vi "generator.vi"() -> ()   [LabVIEW 2013]
panel:
  in  "dzialanie":u16(ring) items=["+", "-", "*", "/", ""]
  in  "z jakim?":u16(ring) items=["noise", "sin", "square", "sawtooth"]
  in  "jaki sygna³?":u16(ring) items=["noise", "sin", "square", "sawtooth"]
  out "wynik dzialania":waveform(dbl)(graph)
  in  "pocz.":dbl
  in  "amplituda":dbl=10.1 caption="Frequency"
  in  "krok":dbl=10.1 caption="Frequency"
  in  "próbkowanie":i32
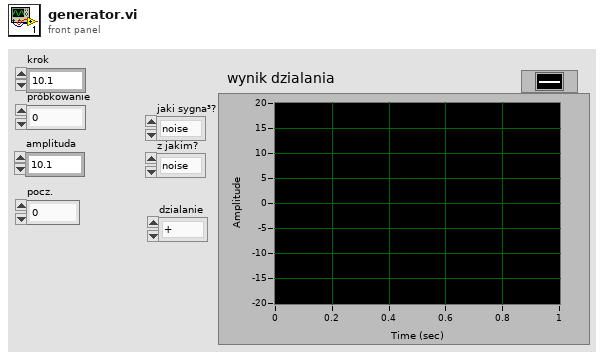
[diagram p1: front panel]
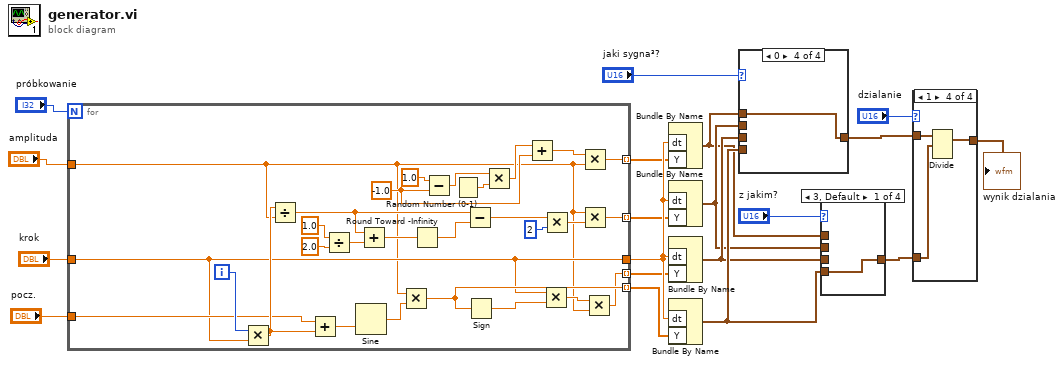
[diagram p0: block diagram]
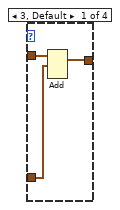
[diagram p2: hidden frame]
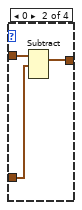
[diagram p3: hidden frame]
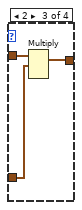
[diagram p4: hidden frame]
diagram:
  n1 = for {
    N: "próbkowanie" -> [_]
    tunnel: [w44] -> w14 mode=indexing
    tunnel: "krok" -> [w25]
    tunnel: [w47] -> w11 mode=indexing
    tunnel: [w21] -> w13 mode=indexing
    tunnel: "amplituda" -> [w20]
    tunnel: [w23] -> w12 mode=indexing
    tunnel: "pocz." -> [w26]
    tunnel: [w25] -> w15
    i -> [w43]
    w42 = -1.0 ("x")
    n2 = Multiply(x=w43, y=w25) -> (x*y=w27:dbl)
    n3 = Divide(x=w27, y=w20) -> (x/y=w34:dbl)
    n4 = Add(x=w26, y=w27) -> (x+y=w28:dbl)
    n5 = Divide(x=1.0, y=2.0) -> (x/y=w31:dbl)
    n6 = Sine(x=w28) -> (sin(x)=w45:dbl)
    n7 = Add(x=w34, y=w31) -> (x+y=w35:dbl)
    n8 = Multiply(x=w20, y=w45) -> (x*y=w44:dbl)
    n9 = Round Toward -Infinity(1:w35) -> (0:w30:dbl)
    n10 = Subtract(x=1.0, y=w42) -> (x-y=w40:dbl)
    n11 = Random Number (0-1)() -> (number: 0 to 1=w39:dbl)
    n12 = Subtract(x=w34, y=w30) -> (x-y=w29:dbl)
    n13 = Sign(1:w44) -> (0:w46:dbl)
    n14 = Multiply(x=w40, y=w39) -> (x*y=w38:dbl)
    n15 = Add(x=w38, y=w42) -> (x+y=w37:dbl)
    n16 = Multiply(x=w25, y=w46) -> (x*y=w22:dbl)
    n17 = Multiply(x=w29, y=2) -> (x*y=w24:dbl)
    n18 = Multiply(x=w37, y=w20) -> (x*y=w47:dbl)
    n19 = Multiply(x=w20, y=w24) -> (x*y=w23:dbl)
    n20 = Multiply(x=w22, y=w20) -> (x*y=w21:dbl)
  }
  n21 = Bundle By Name("dt"=w15, "Y"=w11) -> (w1:waveform(dbl))  [unwired: 1 in]
  n22 = Bundle By Name("dt"=w15, "Y"=w12) -> (w2:waveform(dbl))  [unwired: 1 in]
  n23 = Bundle By Name("dt"=w15, "Y"=w13) -> (w3:waveform(dbl))  [unwired: 1 in]
  n24 = Bundle By Name("dt"=w15, "Y"=w14) -> (w4:waveform(dbl))  [unwired: 1 in]
  n25 = case shown="0" "jaki sygna³?" {
    tunnel: w4 -> [w48 _ _ _]
    tunnel: w3 -> [_ w49 _ _]
    tunnel: w2 -> [_ _ w50 _]
    tunnel: w1 -> [_ _ _ w51]
    tunnel: [w48 w49 w50 w51] -> w10
    frame 3, Default {
    }
    frame 2 {
    }
    frame 1 {
    }
    frame 0 {
    }
  }
  n26 = case shown="3, Default" "z jakim?" {
    tunnel: w4 -> [w52 _ _ _]
    tunnel: w3 -> [_ w53 _ _]
    tunnel: w2 -> [_ _ w54 _]
    tunnel: w1 -> [_ _ _ w55]
    tunnel: [w52 w53 w54 w55] -> w9
    frame 3, Default {
    }
    frame 2 {
    }
    frame 1 {
    }
    frame 0 {
    }
  }
  n27 = case shown="1" "dzialanie" {
    tunnel: w10 -> [w58 w61 w64 w67]
    tunnel: w9 -> [w57 w60 w63 w66]
    tunnel: [w56 w59 w62 w65] -> w8
    frame 3, Default {
      n28 = Add(1:w57, 2:w58) -> (0:w56:waveform(dbl))  [unwired: 1 in, 1 out]
    }
    frame 0 {
      n29 = Subtract(1:w60, 2:w61) -> (0:w59:waveform(dbl))  [unwired: 1 in, 1 out]
    }
    frame 2 {
      n30 = Multiply(1:w63, 2:w64) -> (0:w62:waveform(dbl))  [unwired: 1 in, 1 out]
    }
    frame 1 {
      n31 = Divide(1:w66, 2:w67) -> (0:w65:waveform(dbl))  [unwired: 1 in, 1 out]
    }
  }
  "wynik dzialania" <- w8
